vi "midterm- 2.vi"() -> ()   [LabVIEW 2024]
uses:
  <userlib>/ME121-25-main/ME121-25-main/LabVIEW/SerialVIs/subs/portX.xctl
panel:
  in  "Initial Postion":cluster{"x-position":dbl, "y-position":dbl} {"y-position" scale=0.0..162.5; "x-position" scale=0.0..162.5}
  in  "Final Position":cluster{"x-position":dbl, "y-position":dbl} {"y-position" scale=0.0..162.5; "x-position" scale=0.0..162.5}
  out "Arms":picture
  in  "portX 2":refnum<visa-resource-name>(xcontrol)="ASRL15"
  in  "end effector":cluster{dbl, dbl}={159.01647214211073, 1.9100783062530127} {"?" format="%.1f"; "?" format="%#.1f"}
  in  "L 2":dbl(slide)=85.0 scale=0.0..200.0
  in  "L 1":dbl(slide)=77.5 scale=0.0..200.0
  out "resulting string":string="move(-43,72, -29)"
  # "Advance Dynamics - Midterm - 3DoF Arm"
  # "VI Overview\n\nThis LabVIEW VI controls a 3DoF robotic arm with two links and a chair attached to the end effector. \nThe objective is to move the arm while keeping the chair level to prevent a seated LEGO figure from falling.\nFeatures:\n\n    - Select initial and final positions\n    - Perform inverse kinematics (IK) to compute joint angles\n    - Communicate with a microcontroller to send movement commands\n    - Display a 2D visualization of the arm and its reachable workspace"
  # "1 - Select Port"
  # "User Guide:\n\n    1- Connect to the microcontroller via the port on the right.\n    2 -Select initial and final positions.\n    3 - Click Run:\n       - If the position is within range, a 2D visualization appears, and the user is prompted to execute the                                            \n          movement.\n       -  If out of range, the user is asked to select a valid position.\n\nLet me know if you need further refinements!"
  # "Set an initial position"
  # "mm"
  # "mm"
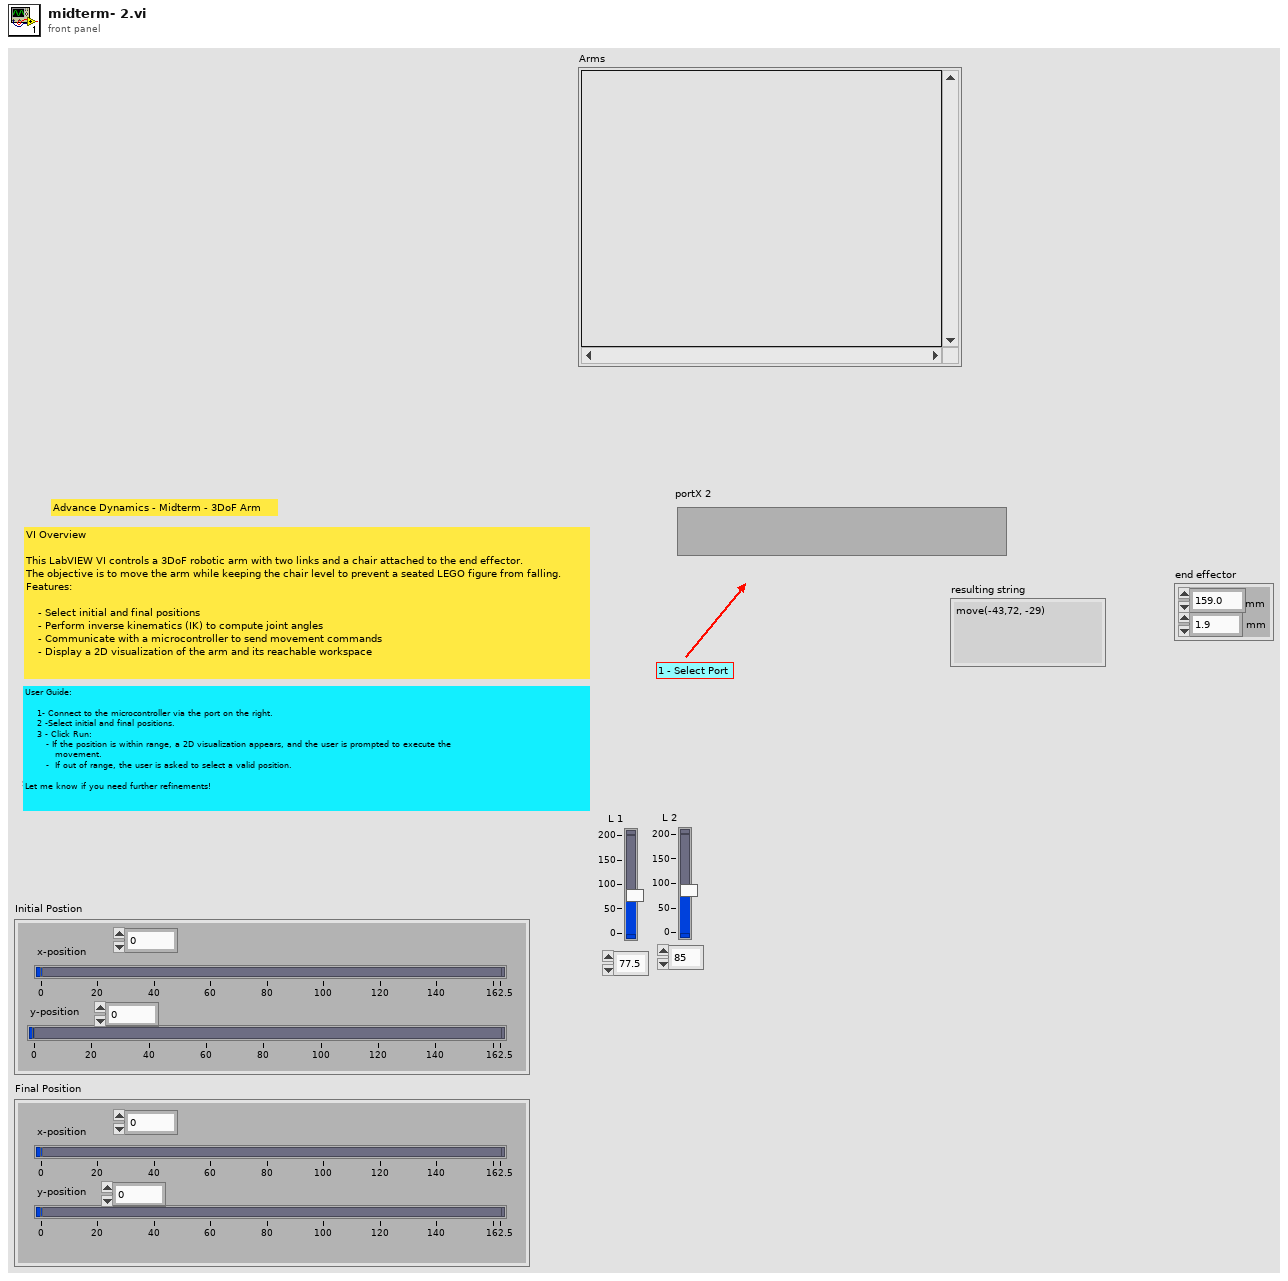
[diagram p1: front panel]
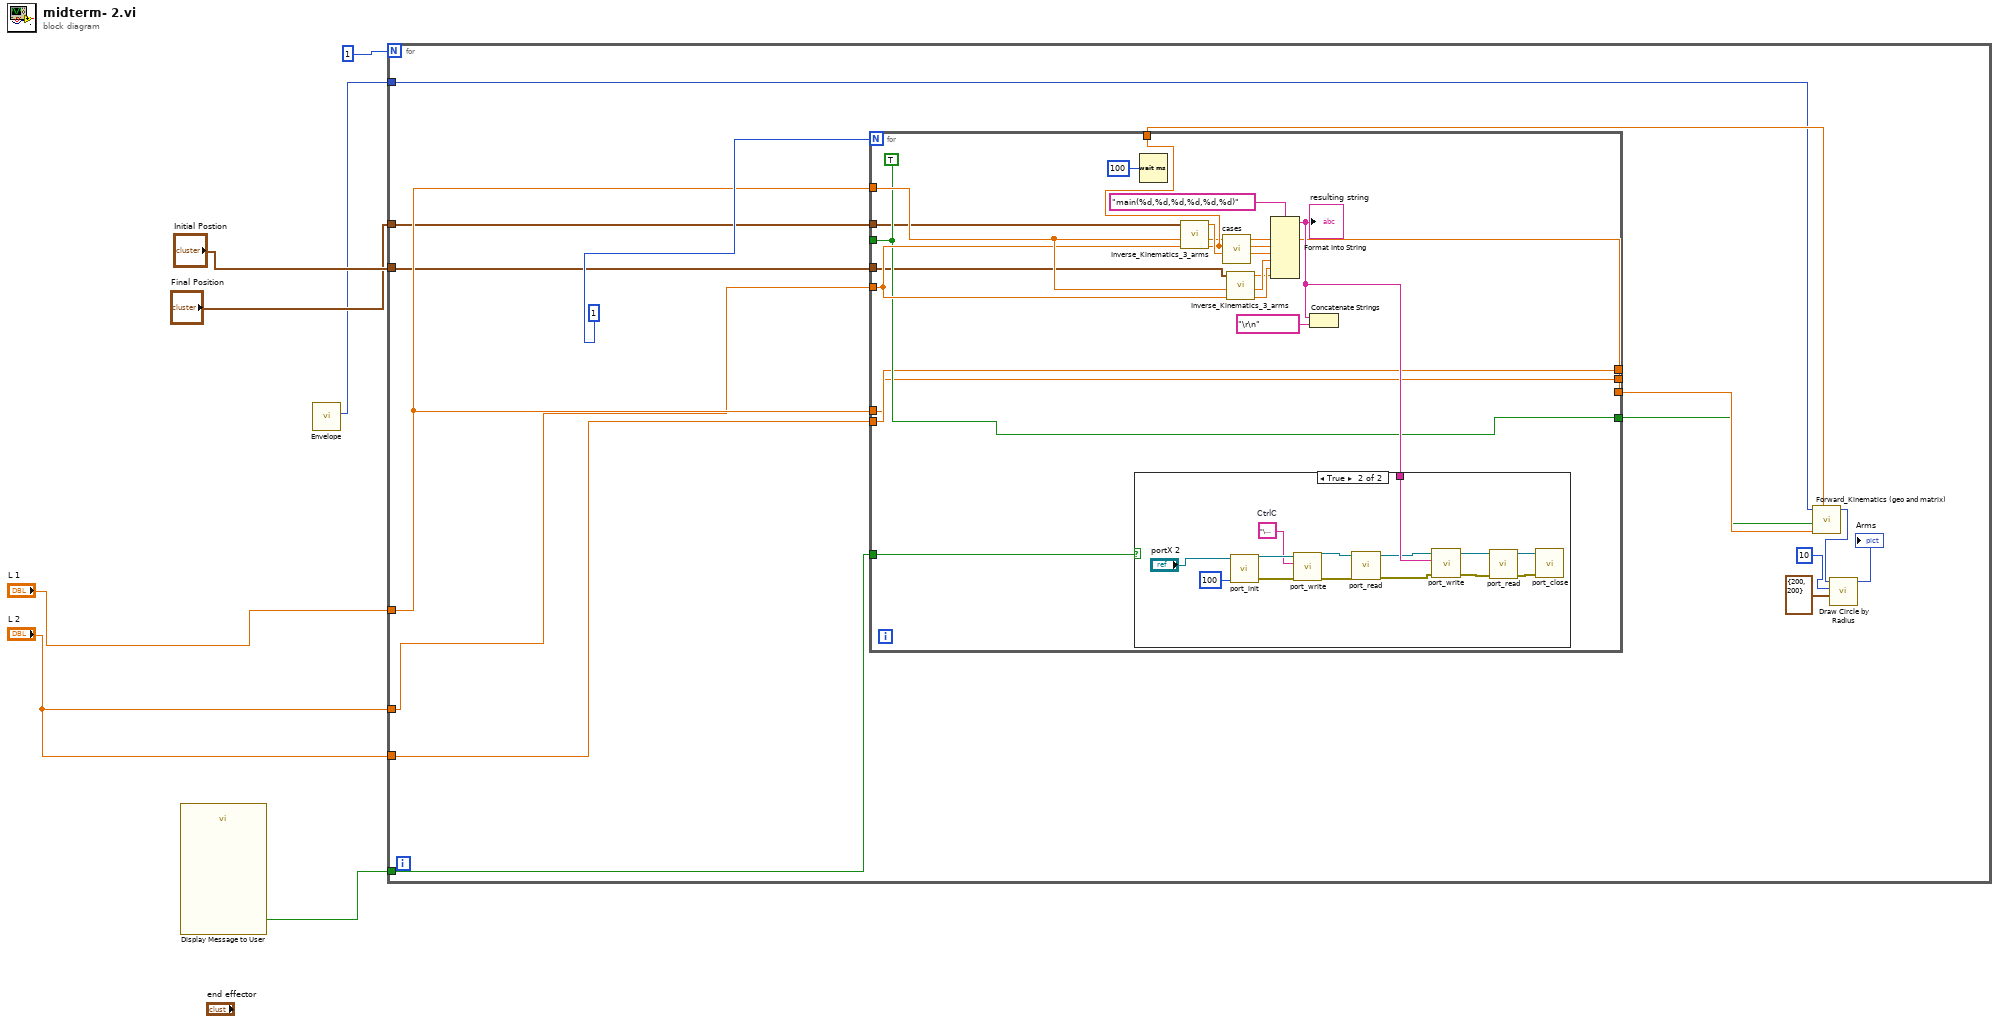
[diagram p0: block diagram]
diagram:
  n1 = call "Display Message to User"() -> ("OK"=w7:bool)  [unwired: 10 in, 1 out]
  n2 = call "Envelope.vi"() -> ("new picture"=w1:picture)  [unwired: 11 in]
  n3 = for {
    N: 1 -> [_]
    tunnel: "L 1" -> [w17]
    tunnel: "L 2" -> [w16]
    tunnel: w7 -> [w15]
    tunnel: "L 2" -> [w14]
    tunnel: "Initial Postion" -> [w10]
    tunnel: "Final Position" -> [w9]
    tunnel: w1 -> [w8]
    n4 = for {
      N: 1 -> [_]
      tunnel: w17 -> [w40]
      tunnel: w16 -> [w30]
      tunnel: [w27] -> _
      tunnel: w15 -> [w31]
      tunnel: w14 -> [w26]
      tunnel: w17 -> [w25]
      tunnel: [w29] -> w13
      tunnel: [w28] -> w12
      tunnel: [w27] -> w11
      tunnel: [w26] -> _
      tunnel: [w25] -> _
      tunnel: w10 -> [w24]
      tunnel: w9 -> [w23]
      w27 = TRUE ("geometry?")
      n5 = Wait (ms)(milliseconds to wait=u32 100) -> ()  [unwired: 1 out]
      n6 = call "Inverse_Kinematics_3_arms.vi"("L 2"=w30, "L 1"=w40, "end effector"=w23) -> ("Angle 2"=w29:dbl, "Angle1"=w28:dbl, "Angle 3"=w32:dbl)  [unwired: 6 in]
      n7 = call "cases.vi"("q 3"=w32, "q 2"=w29, "q 1"=w28) -> ("q3"=w33:dbl, "q2"=w34:dbl, "q1"=w35:dbl)  [unwired: 6 in]
      n8 = call "Inverse_Kinematics_3_arms.vi"("L 2"=w30, "L 1"=w40, "end effector"=w24) -> ("Angle 2"=w38:dbl, "Angle1"=w39:dbl, "Angle 3"=w37:dbl)  [unwired: 6 in]
      n9 = Format Into String(format string="main(%d,%d,%d,%d,%d,%d)", w35, w34, w33, w39, w38, w37) -> (resulting string=w36:string)  [unwired: 2 in, 1 out]
      "resulting string" <- w36
      n10 = case shown="True" w31 {
        tunnel: w36 -> [_ w55]
        frame False {
        }
        frame True {
          w48 = "\u0003"  # CtrlC
          n11 = call <userlib>:"port_init.vi"("Timeout (ms)"=u32 100, "VISA Refnum in"="portX 2") -> ("error out"=w53:errorcluster, "VISA Refnum out"=w54:refnum<visa-resource-name>)  [unwired: 8 in]
          n12 = call <userlib>:"port_write.vi"("error in (no error)"=w53, "write buffer"=w48, "VISA Refnum in"=w54) -> ("error out"=w51:errorcluster, "VISA Refnum out"=w52:refnum<visa-resource-name>)  [unwired: 7 in]
          n13 = call <userlib>:"port_read.vi"("error in (no error)"=w51, "VISA Refnum in"=w52) -> ("error out"=w47:errorcluster, "VISA Refnum out"=w46:refnum<visa-resource-name>)  [unwired: 7 in, 1 out]
          n14 = call <userlib>:"port_write.vi"("error in (no error)"=w47, "write buffer"=w55, "VISA Refnum in"=w46) -> ("error out"=w57:errorcluster, "VISA Refnum out"=w56:refnum<visa-resource-name>)  [unwired: 7 in]
          n15 = call <userlib>:"port_read.vi"("error in (no error)"=w57, "VISA Refnum in"=w56) -> ("error out"=w45:errorcluster, "VISA Refnum out"=w44:refnum<visa-resource-name>)  [unwired: 7 in, 1 out]
          n16 = call <userlib>:"port_close.vi"("error in (no error)"=w45, "VISA Refnum in"=w44) -> ()  [unwired: 10 in]
        }
      }
      n17 = Concatenate Strings(w36, "\r\n") -> ()  [unwired: 1 out]
    }
    n18 = call "Forward_Kinematics (geo and matrix).vi"("q2"=w13, "q1"=w12, "geometry?"=w11, "new picture"=w8) -> ("2D Picture"=w22:picture)  [unwired: 5 in, 2 out]
    n19 = call <vilib>:"Draw Circle by Radius.vi"("pixel center"=cluster{"horizontal":i16, "vertical":i16} {"horizontal"=200, "vertical"=200}, "radius"=i16 10, "picture"=w22) -> ("new picture"=→"Arms":picture)  [unwired: 8 in]
  }
